vi "Intake Arm Controller.vi"(8 "error in":errorcluster) -> ()   [LabVIEW 2020]
doc: "This VI executes continuously carrying out the current operation and responding to updates or new operations. It will often contain the timing or control code that is difficult to place directly in TeleOp. This VI generally opens all sensors and motors and isolates the rest of the robot code from knowing how the operations are carried out."
uses:
  <vilib>/Rock Robotics/WPI/Framework/Completion Status.ctl
  Intake Arm Setpoints.ctl
  Intake Arm Operations.ctl
  <vilib>/Rock Robotics/WPI/Solenoid/WPI_SolenoidValue.ctl
  <vilib>/Rock Robotics/WPI/Solenoid/WPI_SolenoidChannel.ctl
  <vilib>/Rock Robotics/WPI/SafetyOutput/WPI_SafetyOutputConfigMenu.ctl
  <vilib>/Rock Robotics/WPI/Solenoid/WPI_SolenoidOpenDouble.vi
  <vilib>/Rock Robotics/WPI/Solenoid/WPI_SolenoidSetEnum.vi
  <vilib>/Rock Robotics/Network Tables/NT Write Number.vi
panel:
  in  "Interactive Values":T1
  out "Current\nCmd":string
  in  "Buttons":cluster{"Execute Cmd":bool, "Abort Cmd":bool}
  out "Command Timing":cluster{"Start Time (ms)":u32, "Iterations":i32}
  out "Status":T4
  # "Tip: It may be helpful to observe inputs and sensor values.\nYou may also want to display tuning or debugging controls."
  # "Interactive Command: You may fill in the settings for a command\nand schedule it with the Execute button. You can observe and abort\nany command while fine tuning the code for the controller."
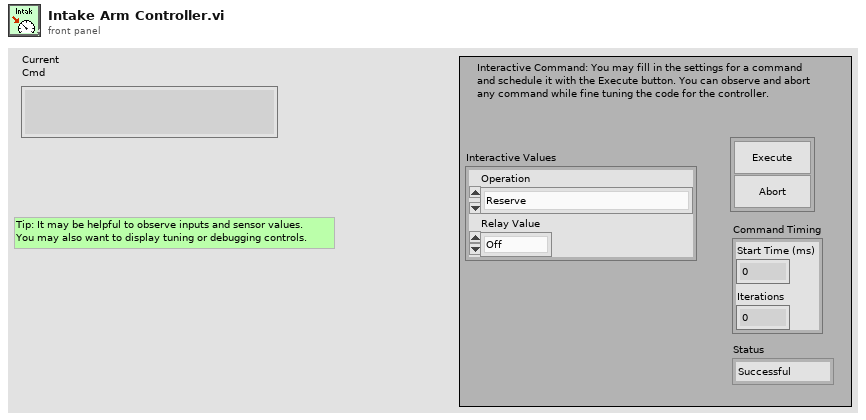
[diagram p1: front panel]
types:
  T1 = typedef "Intake Arm Setpoints.ctl" = cluster{"Operation":T2, "Relay Value":T3}
  T2 = typedef "Intake Arm Operations.ctl" = enum16{"Reserve", "Read Current", "Immediate", "Intake Arm Immediate", "Down", "Up"}
  T3 = typedef "WPI_SolenoidValue.ctl" = enum16{"Off", "On", "Forward", "Reverse"}
  T4 = typedef "Completion Status.ctl" = enum16{"Successful", "Aborted", "Incomplete"}
  T5 = typedef "WPI_SolenoidChannel.ctl" = enum8{"Solenoid 0", "Solenoid 1", "Solenoid 2", "Solenoid 3", "Solenoid 4", "Solenoid 5", "Solenoid 6", "Solenoid 7", "Solenoid 8", "Solenoid 9", "Solenoid 10", "Solenoid 11", "Solenoid 12", "Solenoid 13", "Solenoid 14", "Solenoid 15", "Invalid"}
  T6 = typedef "WPI_SafetyOutputConfigMenu.ctl" = enum16{"Enable", "Disable"}
  T7 = typedef "WPI_SolenoidDevRef.ctl" = cluster{"DevStatus":errorcluster, "Pneumatics Control Module":u8, "Forward Solenoid Channel":T5, "Reverse Solenoid Channel":T5}
  T8 = typedef "Command Status Info.ctl" = cluster{"Name":string, "Status":T4, "notifier out":T9}
  T9 = typedef "Completion Notifier.ctl" = refnum<notifier>
  T10 = cluster{"Current Command":T1, "Command Timing":cluster{"Start Time (ms)":u32, "Iterations":i32}, "Command Arguments":cluster{"Command Info":T8, "Description":string, "Default Command":T1, "queue out":refnum<queue>, "Subsystem Name":string}}
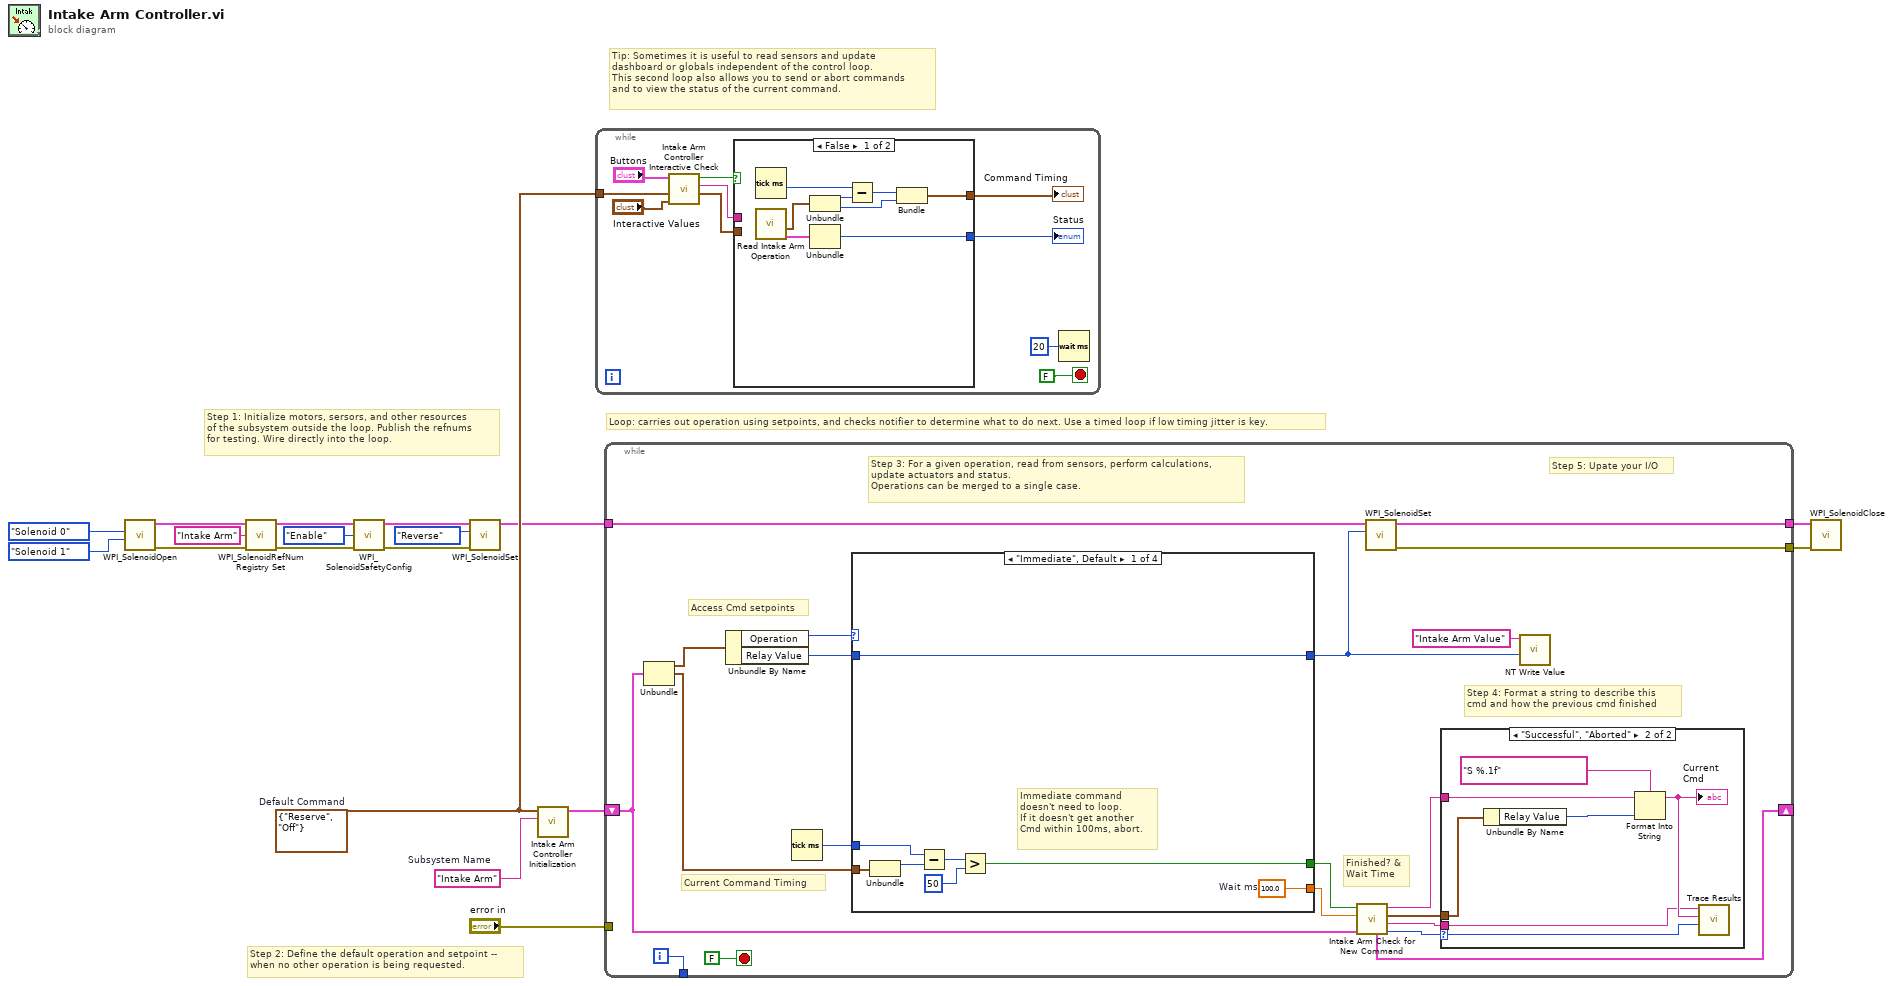
[diagram p0: block diagram]
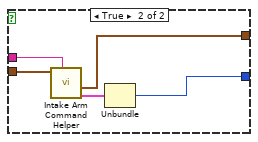
[diagram p2: hidden frame]
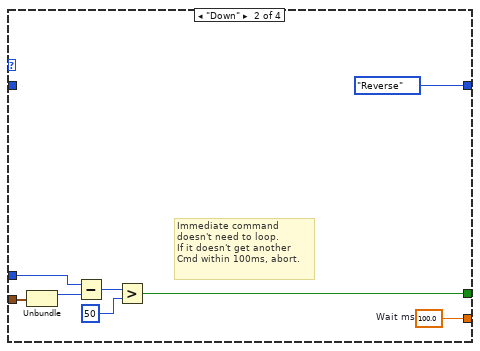
[diagram p4: hidden frame]
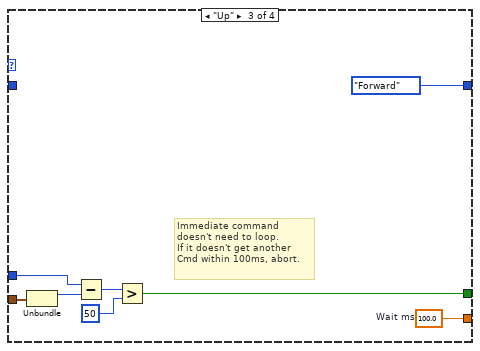
[diagram p5: hidden frame]
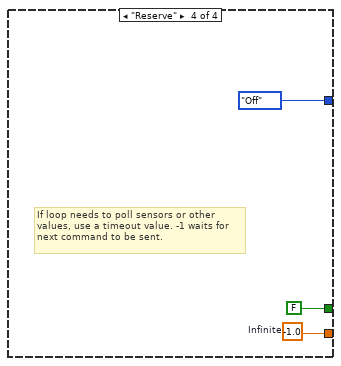
[diagram p6: hidden frame]
diagram:
  w15 = T1 {"Operation"=enum."Reserve", "Relay Value"=enum."Off"}  # Default Command
  w16 = "Intake Arm"  # Subsystem Name
  # "Tip: Sometimes it is useful to read sensors and update\ndashboard or globals independent of the control loop.\nThis second loop also allows you to send or abort commands\nand to view the status of the current command."
  # "Step 2: Define the default operation and setpoint --\nwhen no other operation is being requested."
  # "Step 1: Initialize motors, sersors, and other resources\nof the subsystem outside the loop. Publish the refnums\nfor testing. Wire directly into the loop."
  # "Loop: carries out operation using setpoints, and checks notifier to determine what to do next. Use a timed loop if low timing jitter is key."
  n1 = call-poly <vilib>:"WPI_SolenoidOpen.vi"("Reverse Solenoid Channel"=WPI_SolenoidChannel."Solenoid 1" ("Solenoid Channel"), "Forward Solenoid Channel"=WPI_SolenoidChannel."Solenoid 0" ("Solenoid Channel")) -> ("error out"=w11:errorcluster, "SolenoidDevRef"=w14:T7)  [unwired: 8 in]
  n2 = call <vilib>:"WPI_SolenoidRefNum Registry Set.vi"("error in (no error)"=w11, "refnum name"="Intake Arm", "SolenoidDevRef"=w14) -> ("error out"=w10:errorcluster, "SolenoidDevRef"=w13:T7)  [unwired: 7 in]
  n3 = call <vilib>:"WPI_SolenoidSafetyConfig.vi"("error in (no error)"=w10, "mode"=WPI_SafetyOutputConfigMenu."Enable", "SolenoidDevRef"=w13) -> ("error out"=w9:errorcluster, "SolenoidDevRef"=w12:T7)  [unwired: 7 in]
  n4 = call-poly <vilib>:"WPI_SolenoidSet.vi"("error in (no error)"=w9, "Value"=WPI_SolenoidValue."Reverse", "SolenoidDevRef"=w12) -> ("SolenoidDevRef"=w3:T7)  [unwired: 7 in, 1 out]
  n5 = call "Intake Arm Controller Initialization.vi"("Subsystem Name"=w16, "Default Command"=w15) -> ("Current Command"=w17:T10)  [unwired: 9 in]
  n6 = while {
    tunnel: w15 -> [w25]
    stop <- FALSE stop-if-true
    n7 = call "Intake Arm Controller Interactive Check.vi"("Interactive Command in"="Interactive Values", "Default Command"=w25, "Buttons"="Buttons") -> ("Interactive Command out"=w22:T1, "Trace String"=w23:string, "Schedule"=w24:bool)  [unwired: 6 in]
    n8 = case shown="False" w24 {
      tunnel: [w36 w41] -> w21
      tunnel: w22 -> [_ w39]
      tunnel: [w32 w37] -> w20
      tunnel: w23 -> [_ w40]
      frame False {
        n9 = Tick Count (ms)() -> (millisecond timer value=w31:u32)
        n10 = call "Read Intake Arm Operation.vi"() -> ("Command Info"=w29:T8, "SubSystem Data"=w30:T1)  [unwired: 9 in, 1 out]
        n11 = Unbundle(w30) -> ("Operation"=w35:T2, "Relay Value"=w33:T3)
        n12 = Unbundle(w29) -> ("Status"=w36:T4)  [unwired: 2 out]
        n13 = Subtract(x=w31, y=w35) -> (x-y=w34:u32)
        n14 = Bundle(w34, "Relay Value"=w33) -> (w32:cluster{u32, "Relay Value":T3})  [unwired: 1 in]
      }
      frame True {
        n15 = call "Intake Arm Command Helper.vi"("Description"=w40, "SubSystem Data"=w39) -> ("Command Info Out"=w38:T8, "Command Timing"=w37:cluster{"Start Time (ms)":u32, "Iterations":i32})  [unwired: 7 in, 1 out]
        n16 = Unbundle(w38) -> ("Status"=w41:T4)  [unwired: 2 out]
      }
    }
    "Status" <- w21
    "Command Timing" <- w20
    n17 = Wait (ms)(milliseconds to wait=u32 20) -> ()  [unwired: 1 out]
  }
  n18 = while {
    shift-right: [w55] -> _
    shift-left: w17 -> [w48]
    tunnel: [w60] -> _
    tunnel: "error in" -> [_]
    tunnel: w3 -> [w47]
    tunnel: [w43] -> w2
    tunnel: [w42] -> w1
    i -> [w60]
    stop <- FALSE stop-if-true
    # "Step 5: Upate your I/O"
    # "Step 4: Format a string to describe this\ncmd and how the previous cmd finished"
    # "Current Command Timing"
    # "Access Cmd setpoints"
    # "Finished? &\nWait Time"
    # "Step 3: For a given operation, read from sensors, perform calculations,\nupdate actuators and status.\nOperations can be merged to a single case."
    n19 = Unbundle(w48) -> ("Current Command"=w59:T1, "Command Timing"=w56:cluster{"Start Time (ms)":u32, "Iterations":i32})  [unwired: 1 out]
    n20 = Unbundle By Name(w59) -> ("Operation"=w58:T2, "Relay Value"=w46:T3)
    n21 = Tick Count (ms)() -> (millisecond timer value=w57:u32)
    n22 = case shown="\"Immediate\", Default" w58 {
      tunnel: [w76 w84 w92 w95] -> w53
      tunnel: [w70 w78 w86 FALSE ("ignore previous (F)")] -> w54
      tunnel: w56 -> [w72 w80 w88 _]
      tunnel: w57 -> [w71 w79 w87 _]
      tunnel: [w69 WPI_SolenoidValue."Reverse" ("Value") WPI_SolenoidValue."Forward" ("Value") WPI_SolenoidValue."Off" ("Value")] -> w45
      tunnel: w46 -> [w69 _ _ _]
      frame "Immediate", Default {
        w76 = 100.0  # Wait ms
        # "Immediate command\ndoesn't need to loop.\nIf it doesn't get another\nCmd within 100ms, abort."
        n23 = Unbundle(w72) -> ("Start Time (ms)"=w75:u32)  [unwired: 1 out]
        n24 = Subtract(x=w71, y=w75) -> (x-y=w74:u32)
        n25 = Greater?(x=w74, y=u8 50 ("Left Motor")) -> (0:w70:bool)
      }
      frame "Down" {
        w84 = 100.0  # Wait ms
        # "Immediate command\ndoesn't need to loop.\nIf it doesn't get another\nCmd within 100ms, abort."
        n26 = Unbundle(w80) -> ("Start Time (ms)"=w83:u32)  [unwired: 1 out]
        n27 = Subtract(x=w79, y=w83) -> (x-y=w82:u32)
        n28 = Greater?(x=w82, y=u8 50 ("Left Motor")) -> (0:w78:bool)
      }
      frame "Up" {
        w92 = 100.0  # Wait ms
        # "Immediate command\ndoesn't need to loop.\nIf it doesn't get another\nCmd within 100ms, abort."
        n29 = Unbundle(w88) -> ("Start Time (ms)"=w91:u32)  [unwired: 1 out]
        n30 = Subtract(x=w87, y=w91) -> (x-y=w90:u32)
        n31 = Greater?(x=w90, y=u8 50 ("Left Motor")) -> (0:w86:bool)
      }
      frame "Reserve" {
        w95 = -1.0  # Infinite
        # "If loop needs to poll sensors or other\nvalues, use a timeout value. -1 waits for\nnext command to be sent."
      }
    }
    n32 = call "Intake Arm Check for New Command.vi"("Current Command"=w48, "Wait time (ms)"=w53, "Finished?"=w54) -> ("Completion"=w49:T4, "Subsystem Name"=w50:string, "Current Command"=w51:T1, "Initial Trace String"=w52:string, "NextCommand"=w55:T10)  [unwired: 4 in]
    n33 = call-poly <vilib>:"WPI_SolenoidSet.vi"("Value"=w45, "SolenoidDevRef"=w47) -> ("error out"=w43:errorcluster, "SolenoidDevRef"=w42:T7)  [unwired: 8 in]
    n34 = case shown="\"Successful\", \"Aborted\"" w49 {
      selector: w49 -> [_ w68]
      tunnel: w52 -> [_ w64]
      tunnel: w51 -> [_ w65]
      tunnel: w50 -> [_ w62]
      frame "Incomplete", Default {
        # "Continuing current command"
      }
      frame "Successful", "Aborted" {
        # "Report and setup for next command"
        n35 = Unbundle By Name(w65) -> ("Relay Value"=w67:T3)
        n36 = Format Into String(format string="S %.1f", initial string=w64, w67) -> (resulting string=w63:string)  [unwired: 1 in, 1 out]
        "Current\nCmd" <- w63
        n37 = call <vilib>:"Trace Results.vi"("Status of previous command"=w68, "Description"=w63, "Subsystem"=w62) -> ()  [unwired: 9 in]
      }
    }
    n38 = call-poly <vilib>:"NT Write Value.vi"("Numeric"=w45, "Name"="Intake Arm Value") -> ()  [unwired: 9 in, 1 out]
  }
  n39 = call <vilib>:"WPI_SolenoidClose.vi"("error in (no error)"=w2, "SolenoidDevRef"=w1) -> ()  [unwired: 9 in, 1 out]
